vi "删除零数据.vi"(2 "数组－数值 2":dbl[](array[numeric]), 3 "数组－数值":dbl[](array[numeric])) -> (0 "第二列":dbl[](array[numeric]), 1 "第一列":dbl[](array[numeric]))   [LabVIEW 2016]
panel:
  in  "数组 4":dbl[](array[numeric])
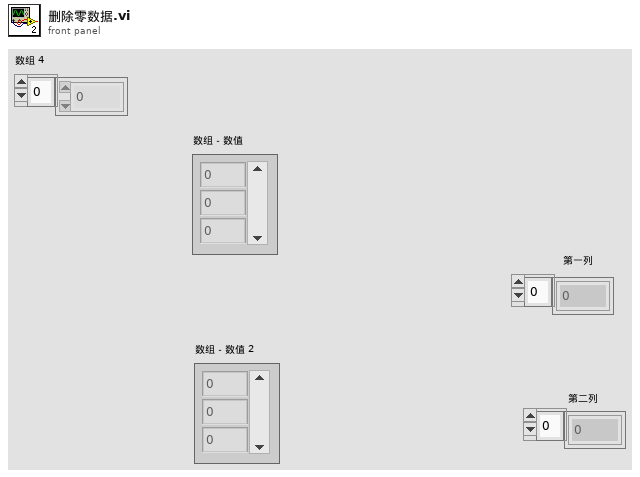
[diagram p1: front panel]
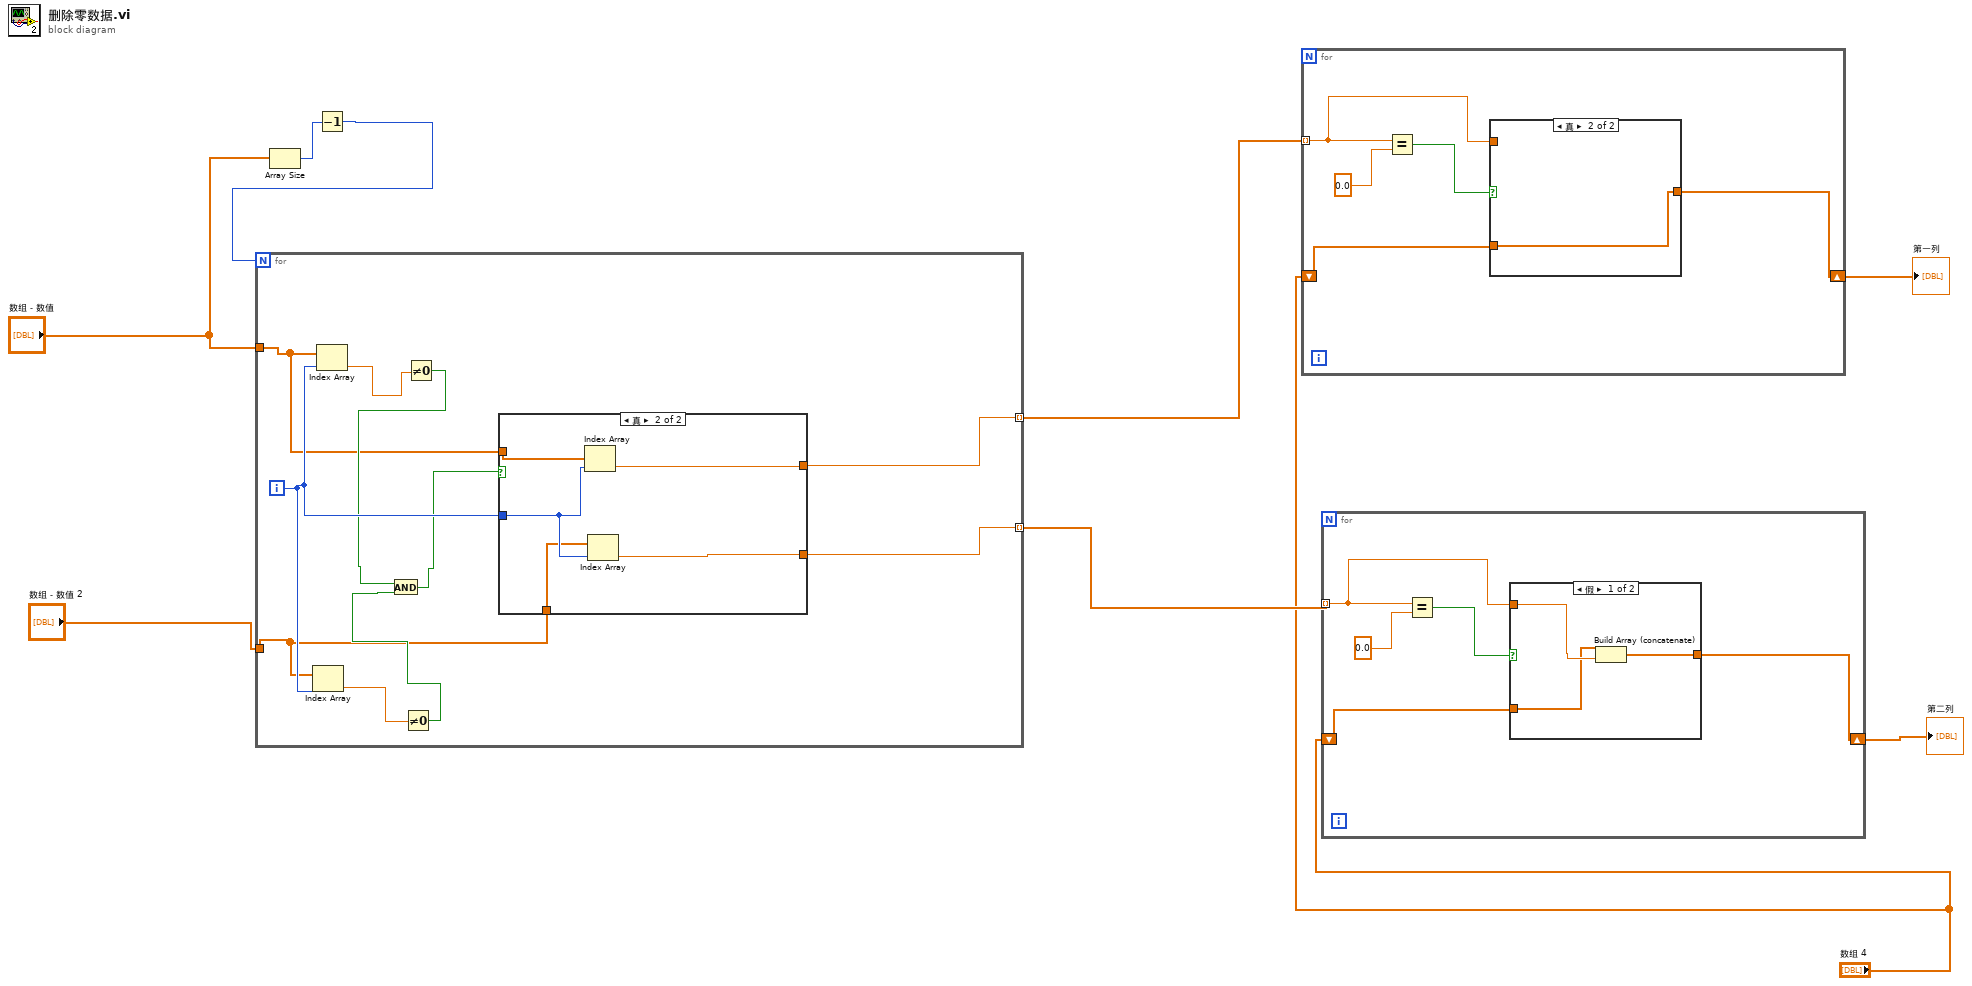
[diagram p0: block diagram]
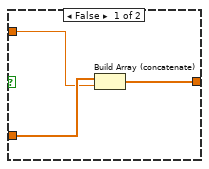
[diagram p3: hidden frame]
diagram:
  n1 = Array Size(array="数组－数值") -> (size(s)=w9:i32)
  n2 = Decrement(x=w9) -> (x-1=w8:i32)
  n3 = for {
    N: w8 -> [_]
    tunnel: [w10] -> w5 mode=indexing
    tunnel: [w13] -> w4 mode=indexing
    tunnel: "数组－数值" -> [w12]
    tunnel: "数组－数值 2" -> [w11]
    i -> [w19]
    n4 = Index Array(array=w11, index=w19) -> (element=w17:dbl)
    n5 = Index Array(array=w12, index=w19) -> (element=w18:dbl)
    n6 = Not Equal To 0?(x=w17) -> (x != 0?=w16:bool)
    n7 = Not Equal To 0?(x=w18) -> (x != 0?=w15:bool)
    n8 = And(x=w15, y=w16) -> (x .and. y?=w14:bool)
    n9 = case shown="真" w14 {
      tunnel: w19 -> [_ w24]
      tunnel: [_ w23] -> w10
      tunnel: [_ w22] -> w13
      tunnel: w12 -> [_ w21]
      tunnel: w11 -> [_ w20]
      frame False {
      }
      frame True {
        n10 = Index Array(array=w21, index=w24) -> (element=w23:dbl)
        n11 = Index Array(array=w20, index=w24) -> (element=w22:dbl)
      }
    }
  }
  n12 = for {
    tunnel: w5 -> [w27] mode=indexing
    shift-right: [w25] -> w2
    shift-left: "数组 4" -> [w26]
    n13 = Equal?(x=w27, y=0.0) -> (x = y?=w28:bool)
    n14 = case shown="真" w28 {
      tunnel: w27 -> [w30 _]
      tunnel: w26 -> [w31 w33]
      tunnel: [w32 w33] -> w25
      frame False {
        n15 = Build Array (concatenate)(w31, w30) -> (w32:dbl[])
      }
      frame True {
      }
    }
  }
  "第一列" <- w2
  n16 = for {
    tunnel: w4 -> [w36] mode=indexing
    shift-right: [w34] -> w1
    shift-left: "数组 4" -> [w35]
    n17 = Equal?(x=w36, y=0.0) -> (x = y?=w37:bool)
    n18 = case shown="假" w37 {
      tunnel: w36 -> [w40 _]
      tunnel: w35 -> [w39 w42]
      tunnel: [w41 w42] -> w34
      frame False {
        n19 = Build Array (concatenate)(w39, w40) -> (w41:dbl[])
      }
      frame True {
      }
    }
  }
  "第二列" <- w1
